vi "Configure.vi"(8 "error in (no error)":errorcluster, 11 "ImageStack in":refnum<class "ImageStack.lvclass">) -> (0 "error out":errorcluster, 2 "cancelled?":bool, 3 "ImageStack out":refnum<class "ImageStack.lvclass">)   [LabVIEW 2012, in "ImageStack.lvclass"]
doc: "The configure method configures the details for the RabbitMQ connection. \n\nIn the derived class, make a call to the parent for setting these parameters."
uses:
  ImageStack.lvclass
  <vilib>/Utility/miscctls.llb/LVPointTypeDef.ctl
  ImageStack.lvclass/ImageStack.ctl
  <vilib>/Distrio/Murmex/Murmex/Murmex.lvclass
panel:
  in  "Cascade name":string
  in  "Orca - Slave name":string
  in  "Orca - Master name":string
  in  "AOTF component name":string
  in  "button:cancel":bool
  in  "button:configure murmex":bool
  in  "button:ok":bool
  in  "Stages component name":string
  in  "Waveform component name":string
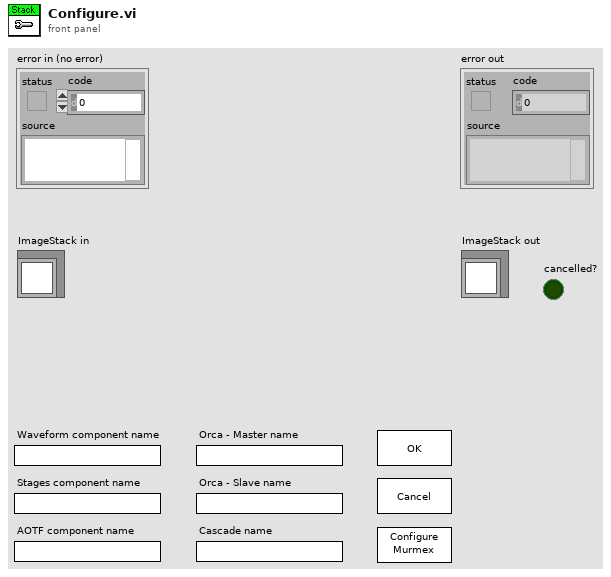
[diagram p1: front panel]
types:
  T1 = typedef "LVPointTypeDef.ctl" = cluster{"Horizontal":i16, "Vertical":i16}
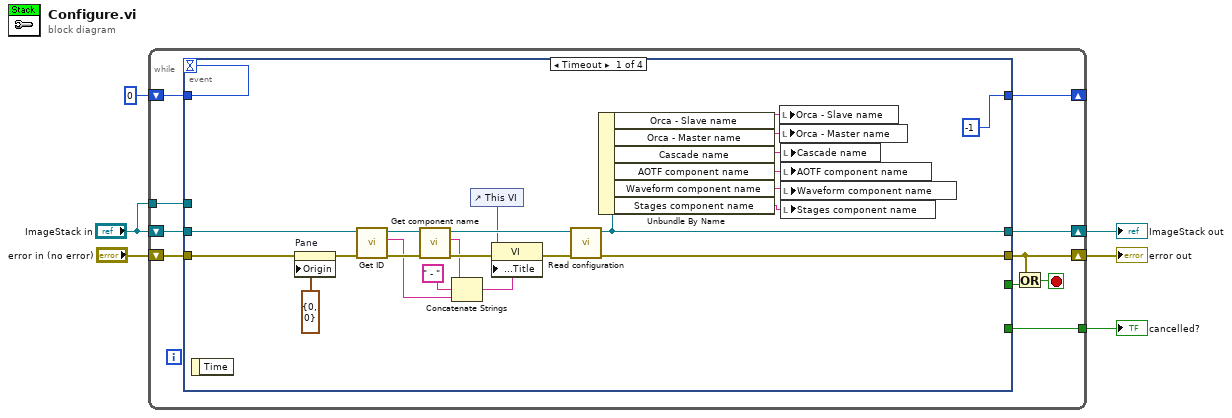
[diagram p0: block diagram]
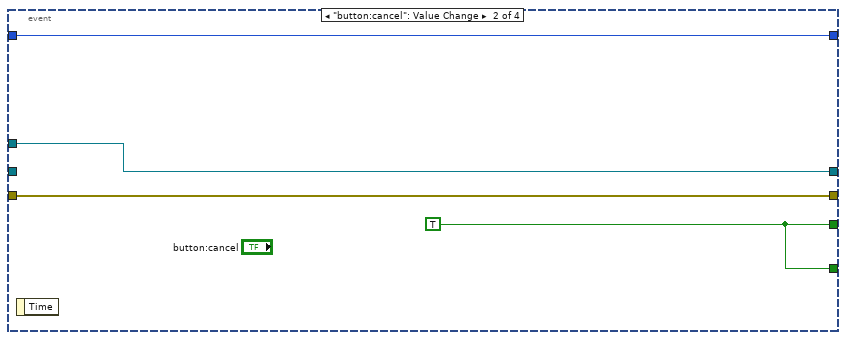
[diagram p2: hidden frame]
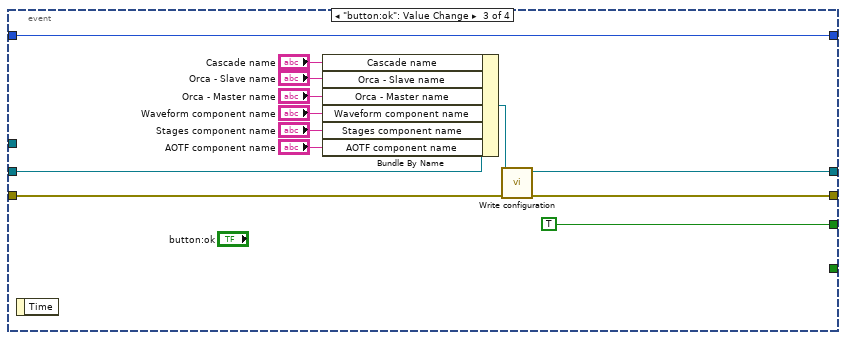
[diagram p3: hidden frame]
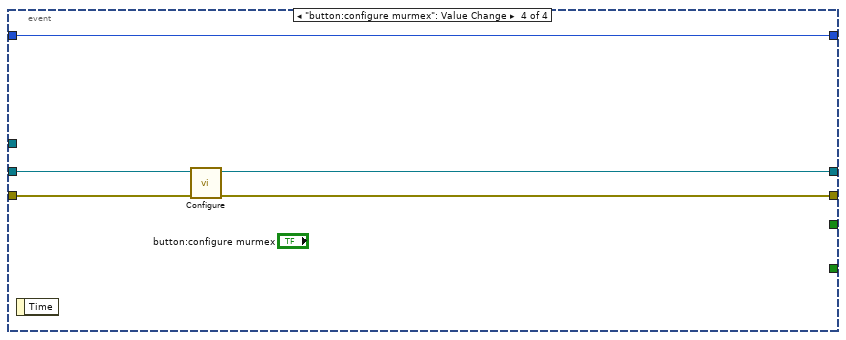
[diagram p4: hidden frame]
diagram:
  n1 = while {
    shift-right: [w11] -> w1
    shift-left: "ImageStack in" -> [w12]
    shift-right: [w13] -> w2
    shift-left: "error in (no error)" -> [w15]
    shift-right: [w16] -> _
    shift-left: 0 -> [w8]
    tunnel: "ImageStack in" -> [w9]
    tunnel: [w7] -> w3
    stop <- w14 stop-if-true
    n2 = event shown="[0] Timeout" {
      selector: _ -> [_ _ _ _]
      dyn-events: _ -> [_ _ _ _]
      timeout: w8 -> [_ _ _ _]
      tunnel: [-1 w41 w48 w57] -> w16
      tunnel: w15 -> [w37 w43 w52 w60]
      tunnel: [w38 w43 w50 w58] -> w13
      tunnel: w12 -> [w34 _ w56 w61]
      tunnel: [w23 w42 w51 w59] -> w11
      tunnel: [_ w40 TRUE _] -> w10
      tunnel: w9 -> [_ w42 _ _]
      tunnel: w8 -> [_ w41 w48 w57]
      tunnel: [_ w40 _ _] -> w7
      event Timeout {
        n3 = event-data() -> ()  [unwired: 1 in, 1 out]
        n4 = property on="Pane" class="Pane"(error in=w37, "Origin"=T1 {"Horizontal"=0, "Vertical"=0}) -> (error out=w35:errorcluster)  [unwired: 1 in, 1 out]
        n5 = call <vilib>:"Get ID.vi"("error in (no error)"=w35, "Murmex in"=w34) -> ("error out"=w32:errorcluster, "component id"=w28:string, "Murmex out"=w33:refnum<class "ImageStack.lvclass">)  [unwired: 7 in]
        n6 = call <vilib>:"Get component name.vi"("error in (no error)"=w32, "Murmex in"=w33) -> ("error out"=w31:errorcluster, "component name"=w29:string, "Murmex out"=w30:refnum<class "ImageStack.lvclass">)  [unwired: 7 in]
        n7 = Concatenate Strings(w29, " - " ("element"), w28) -> (w24:string)
        n8 = control-ref of="This VI"() -> (w25:refnum<vi>)
        n9 = property class="VI"(reference=w25, error in=w31, "Front Panel.Title"=w24) -> (error out=w26:errorcluster)  [unwired: 1 out]
        n10 = call <vilib>:"Read configuration.vi"("error in (no error)"=w26, "Murmex in"=w30) -> ("error out"=w38:errorcluster, "Murmex out"=w23:refnum<class "ImageStack.lvclass">)  [unwired: 7 in, 1 out]
        n11 = Unbundle By Name(w23) -> ("Orca - Slave name"=w17:string, "Orca - Master name"=w18:string, "Cascade name"=w19:string, "AOTF component name"=w20:string, "Waveform component name"=w22:string, "Stages component name"=w21:string)
        n12 = local write "Orca - Slave name"(w17) -> ()
        n13 = local write "Orca - Master name"(w18) -> ()
        n14 = local write "Cascade name"(w19) -> ()
        n15 = local write "AOTF component name"(w20) -> ()
        n16 = local write "Waveform component name"(w22) -> ()
        n17 = local write "Stages component name"(w21) -> ()
      }
      event "button:cancel": Value Change {
        w40 = TRUE
        n18 = event-data() -> ()  [unwired: 1 in, 1 out]
      }
      event "button:ok": Value Change {
        n19 = event-data() -> ()  [unwired: 1 in, 1 out]
        n20 = Bundle By Name(cluster=w56, "Cascade name"="Cascade name", "Orca - Slave name"="Orca - Slave name", "Orca - Master name"="Orca - Master name", "Waveform component name"="Waveform component name", "Stages component name"="Stages component name", "AOTF component name"="AOTF component name") -> (w55:refnum<class "ImageStack.lvclass">)
        n21 = call <vilib>:"Write configuration.vi"("error in (no error)"=w52, "Murmex in"=w55) -> ("error out"=w50:errorcluster, "Murmex out"=w51:refnum<class "ImageStack.lvclass">)  [unwired: 8 in]
      }
      event "button:configure murmex": Value Change {
        n22 = event-data() -> ()  [unwired: 1 in, 1 out]
        n23 = call-parent "Configure.vi"("error in (no error)"=w60, "Murmex in"=w61) -> ("error out"=w58:errorcluster, "Murmex out"=w59:refnum<class "ImageStack.lvclass">)  [unwired: 7 in, 1 out]
      }
    }
    n24 = Or(x=w13, y=w10) -> (x .or. y?=w14:bool)
  }
  "error out" <- w2
  "ImageStack out" <- w1
  "cancelled?" <- w3
